vi "Set Class.vi"(8 "error in (no error)":errorcluster caption="错误输入（无错误）", 9 "项标识符":string, 10 "LNK.lvclass":refnum<class "Menu.lvclass">, 11 "listbox 输入":refnum<class "listbox.lvclass">) -> (0 "error out":errorcluster caption="错误输出", 3 "listbox 输出":refnum<class "listbox.lvclass">)   [LabVIEW 2016, in "listbox.lvclass"]
uses:
  listbox.lvclass
  LNK/Parent Class/Menu.lvclass
  listbox.lvclass/listbox.ctl
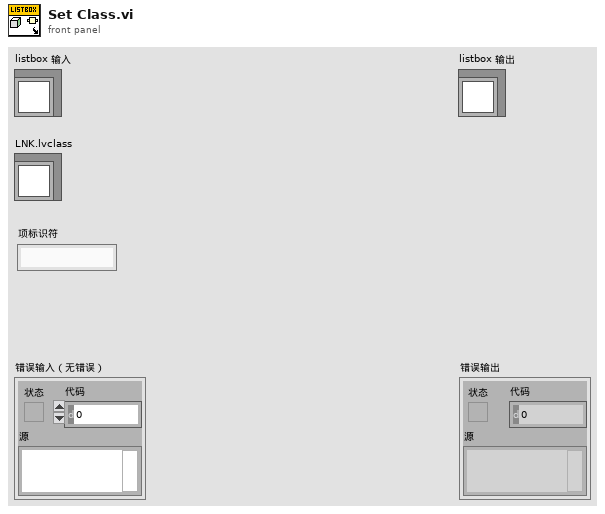
[diagram p1: front panel]
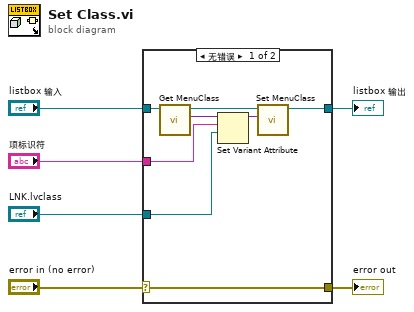
[diagram p0: block diagram]
diagram:
  n1 = case shown="无错误" "error in (no error)" {
    selector: "error in (no error)" -> [w13 w16]
    tunnel: [w13 w16] -> w5
    tunnel: [w11 w15] -> w3
    tunnel: "listbox 输入" -> [w14 w15]
    tunnel: "项标识符" -> [w8 _]
    tunnel: "LNK.lvclass" -> [w7 _]
    frame No Error {
      n2 = call "Get MenuClass.vi"("listbox in"=w14) -> ("MenuClass"=w10:variant, "listbox out"=w12:refnum<class "listbox.lvclass">)  [unwired: 9 in]
      n3 = Set Variant Attribute(Variant=w10, name=w8, value=w7) -> (Variant out=w9:variant)  [unwired: 1 in, 2 out]
      n4 = call "Set MenuClass.vi"("MenuClass"=w9, "listbox in"=w12) -> ("listbox out"=w11:refnum<class "listbox.lvclass">)  [unwired: 9 in]
    }
    frame Error {
    }
  }
  "error out" <- w5
  "listbox 输出" <- w3
